vi "FTW-Test-JSON-Fuzz.vi"() -> (0 "Test Result":errorcluster)   [LabVIEW 2015]
uses:
  codegen/xnode/FTW-Dataflow-Synchronizer.xnode
panel:
  out "JSON String (UTF-8)":string
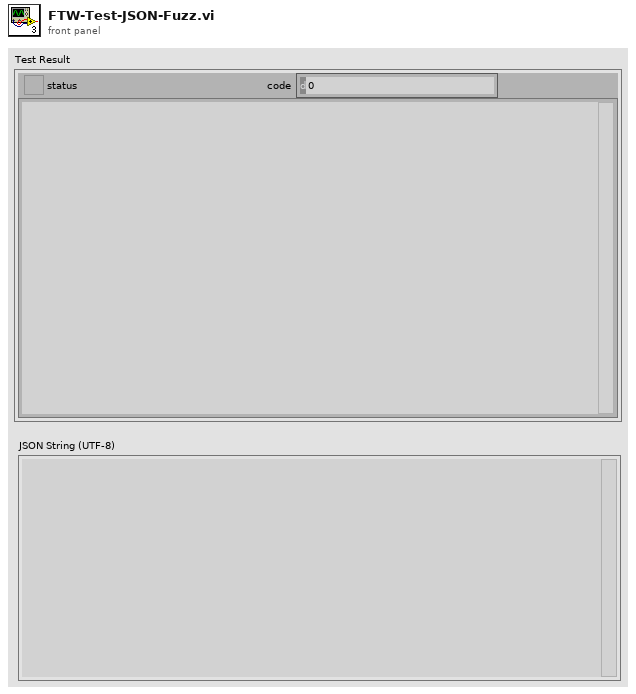
[diagram p1: front panel]
types:
  T1 = typedef "FTW-Type-JSON.ctl" = refnum<data-value>
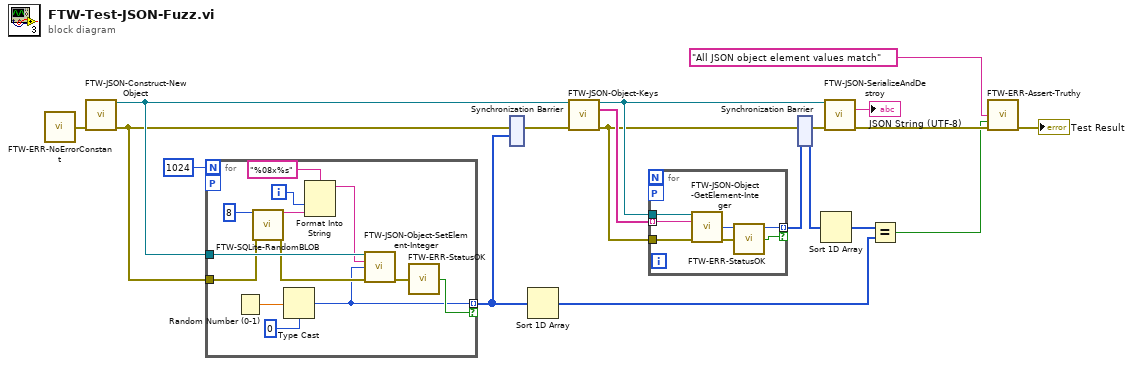
[diagram p0: block diagram]
diagram:
  n1 = call "FTW-ERR-NoErrorConstant.vi"() -> ("no error"=w16:errorcluster)
  n2 = call "FTW-JSON-Construct-NewObject.vi"("error in"=w16) -> ("JSON"=w18:refnum<class "FTW-Container.lvclass">, "error out"=w7:errorcluster)  [unwired: 13 in]
  n3 = for {
    N: 1024 -> [_]
    workers-P: _ -> [_]
    tunnel: w7 -> [w30]
    tunnel: w18 -> [w32]
    tunnel: [w21] -> w5 mode=indexing if=w23
    i -> [w26]
    n4 = Random Number (0-1)() -> (number: 0 to 1=w22:dbl)
    n5 = call "FTW-SQLite-RandomBLOB.vi"("Number of Bytes"=8, "error in"=w30) -> ("Random BLOB"=w27:string, "error out"=w29:errorcluster)  [unwired: 12 in]
    n6 = Type Cast(type=i64 0, x=w22) -> (*(type *) &x=w21:i64)
    n7 = Format Into String(format string="%08x%s", w26, w27) -> (resulting string=w24:string)  [unwired: 2 in, 1 out]
    n8 = call "FTW-JSON-Object-SetElement-Integer.vi"("JSON"=w32, "Key"=w24, "Value"=w21, "error in"=w29) -> ("error out"=w28:errorcluster)  [unwired: 10 in, 1 out]
    n9 = call "FTW-ERR-StatusOK.vi"("error to check"=w28) -> ("Status OK?"=w23:bool)
  }
  n10 = xnode "Synchronization Barrier"("Synchronized Signal 1"=w7, "Synchronized Signal 2"=w5) -> ("error out out"=w6:errorcluster)  [unwired: 1 out]
  n11 = Sort 1D Array(array=w5) -> (sorted array=w13:i64[])
  n12 = call "FTW-JSON-Object-Keys.vi"("JSON"=w18, "error in"=w6) -> ("JSON out"=w11:T1, "Keys"=w15:string[], "error out"=w2:errorcluster)  [unwired: 11 in]
  n13 = for {
    tunnel: w15 -> [w37] mode=indexing
    tunnel: [w35] -> w4 mode=indexing if=w33
    workers-P: _ -> [_]
    tunnel: w11 -> [w38]
    tunnel: w2 -> [w36]
    n14 = call "FTW-JSON-Object-GetElement-Integer.vi"("JSON"=w38, "Key"=w37, "error in"=w36) -> ("Value"=w35:i64, "error out"=w34:errorcluster)  [unwired: 9 in, 2 out]
    n15 = call "FTW-ERR-StatusOK.vi"("error to check"=w34) -> ("Status OK?"=w33:bool)
  }
  n16 = xnode "Synchronization Barrier"("Synchronized Signal 1"=w2, "Synchronized Signal 2"=w4) -> ("error out out"=w1:errorcluster, "out"=w3:i64[])
  n17 = Sort 1D Array(array=w3) -> (sorted array=w14:i64[])
  n18 = call "FTW-JSON-SerializeAndDestroy.vi"("JSON"=w11, "error in"=w1) -> ("JSON String (UTF-8)"=→"JSON String (UTF-8)":string, "error out"=w10:errorcluster)  [unwired: 12 in]
  n19 = Equal?(x=w14, y=w13) -> (x = y?=w9:bool)
  n20 = call "FTW-ERR-Assert-Truthy.vi"("Assertion"="All JSON object element values match", "Assertion holds true?"=w9, "error in"=w10) -> ("error out"=→"Test Result":errorcluster)  [unwired: 12 in]
